vi "Calculator_Calculator-harness.vi"(11 "test case ID":string) -> (3 "result":bool)   [LabVIEW 2020]
doc: "The harness VI is executed for every test case. InstaCoverage passes the test case ID before the execution of the test case in the <b>test case ID</b> input and reads the <b>result</b> output after the execution. If the result is TRUE and no error happens during the execution, then the test case is evaluated as PASSED. If the result is false and no error happens during the execution, then the test case is evaluated as FAILED. Otherwise the test case is evaluated as ERROR.\n\nThe result of the test suite will be PASSED (FAILED) if all (at least one) test cases are PASSED (FAILED). If at least one test case in the test suite has the ERROR result, then the test suite will have ERROR result.\n\n<b>Note: </b>Don't change the connector pane of this VI.\n\nSee the Help Document for more information. (<b>Help</b> > <b>InstaCoverage Help...</b>)"
uses:
  LabVIEW Data/Calculator/Calculator.lvclass
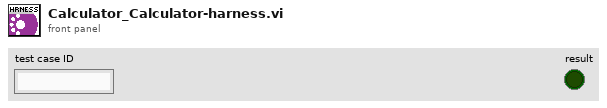
[diagram p1: front panel]
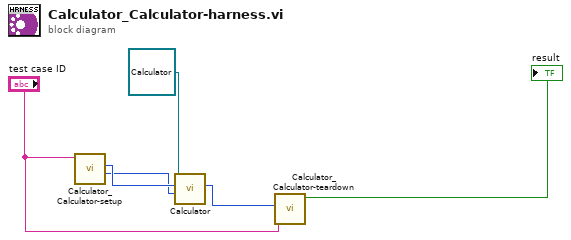
[diagram p0: block diagram]
diagram:
  n1 = call "Calculator_Calculator-setup.vi"("test case ID"="test case ID") -> ("Numeric 2"=w2:i32, "Numeric"=w3:i32)  [unwired: 9 in]
  n2 = call "Calculator.vi"("Input 2"=w2, "Input 1"=w3, "Calculator in"=refnum<class "Calculator.lvclass"> refnum) -> ("Output"=w1:i32)  [unwired: 6 in, 2 out]
  n3 = call "Calculator_Calculator-teardown.vi"("Numeric"=w1, "test case ID"="test case ID") -> ("result"=→"result":bool)  [unwired: 9 in]
